vi "Robot Auto Drive.vi"(8 "Time (ms)":u32, 9 "X axis value":dbl, 10 "Y axis value":dbl, 11 "RobotDriveDevRef":T1) -> (3 "RobotDriveDevRef Out":T1={"DevStatus"={"status"=FALSE, "code"=0, "source"=""}, "Motors[]"=[], "Square Inputs"=FALSE, "Max Output"=1.0})   [LabVIEW 2019]
uses:
  <vilib>/Rock Robotics/WPI/RobotDrive/WPI_RobotDriveDevRef.ctl
  <vilib>/Rock Robotics/WPI/MotorControl/WPI_MotorControlDeviceRef.ctl
  <vilib>/Rock Robotics/WPI/MotorControl/WPI_MotorControlType.ctl
  <vilib>/Rock Robotics/SystemInterfaces/DIO/FPGA_DIOPWMChannel.ctl
  <vilib>/Rock Robotics/WPI/PWM/WPI_PWMDeadband.ctl
  <vilib>/Rock Robotics/SystemInterfaces/DIO/FPGA_DIOChannel.ctl
  <vilib>/Rock Robotics/WPI/RobotDrive/WPI_RobotDriveArcadeDrive_Standard(NoSaturation).vi
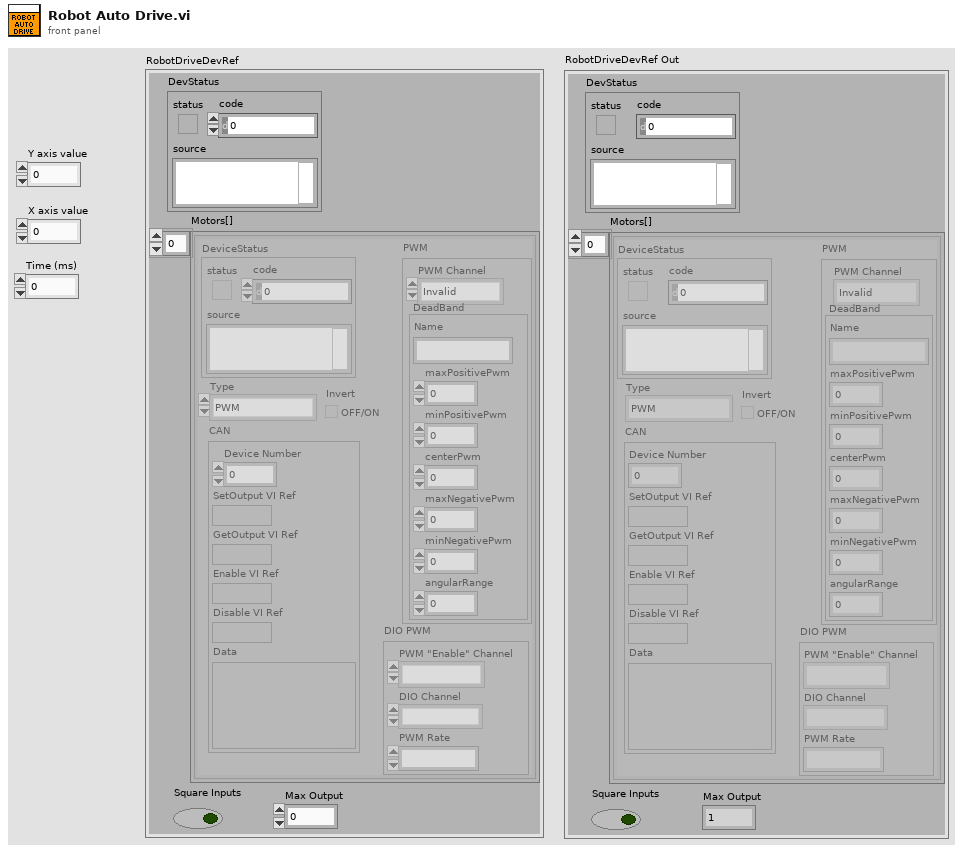
[diagram p1: front panel]
types:
  T1 = typedef "WPI_RobotDriveDevRef.ctl" = cluster{"DevStatus":errorcluster, "Motors[]":T2[], "Square Inputs":bool, "Max Output":dbl}
  T2 = typedef "WPI_MotorControlDeviceRef.ctl" = cluster{"DeviceStatus":errorcluster, "Type":T3, "PWM":cluster{"PWM Channel":T4, "DeadBand":T5}, "CAN":cluster{"Device Number":u8, "SetOutput VI Ref":variant, "GetOutput VI Ref":variant, "Enable VI Ref":variant, "Disable VI Ref":variant, "Data":variant}, "Invert":bool, "DIO PWM":cluster{"PWM \"Enable\" Channel":T4, "DIOChannel":T6, "PWM Rate":dbl}}
  T3 = typedef "WPI_MotorControlType.ctl" = enum16{"PWM", "CAN", "DIO PWM"}
  T4 = typedef "FPGA_DIOPWMChannel.ctl" = enum8{"PWM 0", "PWM 1", "PWM 2", "PWM 3", "PWM 4", "PWM 5", "PWM 6", "PWM 7", "PWM 8", "PWM 9", "PWM MXP 0", "PWM MXP 1", "PWM MXP 2", "PWM MXP 3", "PWM MXP 4", "PWM MXP 5", "PWM MXP 6", "PWM MXP 7", "PWM MXP 8", "PWM MXP 9", "Invalid"}
  T5 = typedef "WPI_PWMDeadband.ctl" = cluster{"Name":string, "maxPositivePwm":i32, "minPositivePwm":i32, "centerPwm":i32, "maxNegativePwm":i32, "minNegativePwm":i32, "angularRange":u16}
  T6 = typedef "FPGA_DIOChannel.ctl" = enum8{"DIO 0", "DIO 1", "DIO 2", "DIO 3", "DIO 4", "DIO 5", "DIO 6", "DIO 7", "DIO 8", "DIO 9", "DIO MXP 0", "DIO MXP 1", "DIO MXP 2", "DIO MXP 3", "DIO MXP 4", "DIO MXP 5", "DIO MXP 6", "DIO MXP 7", "DIO MXP 8", "DIO MXP 9", "DIO MXP 10", "DIO MXP 11", "DIO MXP 12", "DIO MXP 13", "DIO MXP 14", "DIO MXP 15", "SPI Port CS1", "SPI Port CS2", "SPI Port CS3", "SPI Port MISO", "SPI Port MOSI", "Invalid"}
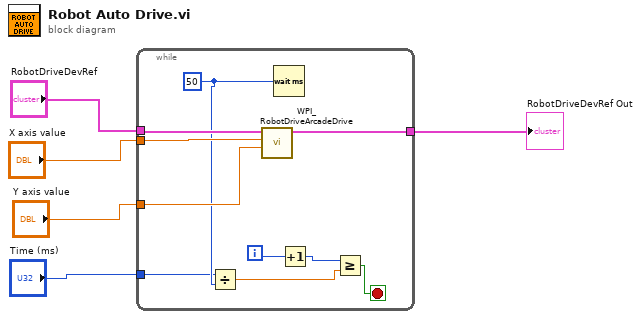
[diagram p0: block diagram]
diagram:
  n1 = while {
    tunnel: "RobotDriveDevRef" -> [w15]
    tunnel: "X axis value" -> [w14]
    tunnel: "Y axis value" -> [w13]
    tunnel: "Time (ms)" -> [w7]
    tunnel: [w6] -> w1
    i -> [w12]
    stop <- w10 stop-if-true
    w8 = u32 50 ("milliseconds to wait")
    n2 = Divide(x=w7, y=w8) -> (x/y=w9:dbl)
    n3 = call-poly <vilib>:"WPI_RobotDriveArcadeDrive.vi"("Y axis value"=w13, "X axis value"=w14, "RobotDriveDevRef"=w15) -> ("RobotDriveDevRef"=w6:T1)  [unwired: 6 in, 2 out]
    n4 = Wait (ms)(milliseconds to wait=w8) -> ()  [unwired: 1 out]
    n5 = Increment(x=w12) -> (x+1=w11:i32)
    n6 = Greater Or Equal?(x=w11, y=w9) -> (x >= y?=w10:bool)
  }
  "RobotDriveDevRef Out" <- w1
